vi "Measurement Logic.vi"() -> ()   [LabVIEW 2021, in "Single Tone Measurements_Class D Amplifier.lvlib"]
uses:
  Single Tone Measurements_Class D Amplifier.lvlib
  Measurement Configuration.ctl
  shared/controls/digital audio protocol/data justification.ctl
  shared/controls/digital audio protocol/endianness.ctl
  shared/controls/digital audio protocol/digital edge.ctl
  shared/controls/digital audio protocol/logic level.ctl
  shared/controls/output mode.ctl
  shared/controls/weighting filter.ctl
  shared/controls/lowpass filter.ctl
  shared/controls/highpass filter.ctl
  shared/controls/units - snr.ctl
  shared/controls/units - ratio.ctl
  Measurement Results.ctl
  <vilib>/MeasurementLink/MeasurementLink Measurement Server/Classes/MeasurementContext/MeasurementContext.lvclass
  shared/controls/single tone audio measurements.ctl
  <vilib>/PDM Acquisition Toolkit/shared/controls/clock mode.ctl
  <vilib>/PDM Acquisition Toolkit/shared/controls/PCM Frame Sync Control.ctl
  <vilib>/PDM Acquisition Toolkit/shared/controls/Digital Edge.ctl
  <vilib>/PDM Acquisition Toolkit/shared/controls/PCM Data Format Configuration.ctl
  <vilib>/PDM Acquisition Toolkit/shared/controls/PCM Bit Endianness.ctl
  <vilib>/PDM Acquisition Toolkit/shared/controls/PCM Data Justification.ctl
  shared/controls/single tone audio measurement settings.ctl
  shared/controls/audio filter settings.ctl
  shared/controls/units settings.ctl
  <vilib>/DAQmx/read.llb/DAQmx Read (Analog 1D Wfm NChan NSamp).vi
  <vilib>/PDM Acquisition Toolkit/host/API/Public/Function Generator/Configure Custom Signal (N Ch) - PCM Output Task.vi
  <vilib>/DAQmx/create/channels.llb/DAQmx Create Channel (AI-Voltage-Basic).vi
  <vilib>/DAQmx/configure/timing.llb/DAQmx Timing (Sample Clock).vi
  <vilib>/DAQmx/miscellaneous.llb/DAQmx Fill In Error Info.vi
  <vilib>/Waveform/WDTOps.llb/WDT Get Waveform Subset DBL.vi
  <vilib>/PDM Acquisition Toolkit/shared/PDM Shared.lvlib
  <vilib>/PDM Acquisition Toolkit/host/API/PDM Acquisition Toolkit.lvlib
  shared/controls/audio controls.lvlib
  shared/controls/digital audio protocol/digital audio protocol controls.lvlib
panel:
  out "results":T1={"channel"="0", "frequency (Hz)"=1000.0000024177915, "amplitude (Vrms)"=-6.256665451281146, "amplitude (dBFS)"=0.0, "SNR"=78.42395339546047, "THD+N"=-71.07176133726693, "THD"=-71.98384642729017, "dynamic range (dB)"=83.34902670182771, "gain"=-0.25666545128114626, "SFDR (dBc)"=102.93430172121762}
  out "Spectrum":cluster{"x0":dbl, "dx":dbl, "magnitude":dbl[]}(graph)={"x0"=0.0, "dx"=4.000000000559116, "magnitude"=array[6400 elements]}
  out "Waveform Graph":waveform(dbl)[](graph)=[{"t0"=timestamp(3785336549.595634 s since 1904-01-01), "dt"=1.9531249997269942e-05, "Y"=array[12800 elements], "attributes"=variant("NI_ChannelName"=variant(string "PXI1Slot4/ai0"), "NI_UnitDescription"=variant(string "Volts"))}]
  out "Bit Clock Rate":sgl=3072000.0 format="%#_6pHz"
  out "Measurement Context out":refnum<class "MeasurementContext.lvclass">
  in  "Measurement Context":refnum<class "MeasurementContext.lvclass">=refnum
  out "Measurement Results":T2={"channel name"="0", "frequency (Hz)"=1000.0000024177915, "amplitude (Vrms)"=-6.256665451281146, "amplitude (dBFS)"=0.0, "SNR"=78.42395339546047, "THD+N"=-71.07176133726693, "THD"=-71.98384642729017, "dynamic range (dB)"=83.34902670182771, "gain"=-0.25666545128114626, "SFDR (dBc)"=102.93430172121762, "output power (W)"=0.0, "wfm - t0"=0.0, "wfm - dt"=1.9531249997269942e-05, "wfm - data"=array[12800 elements], "fft - f0"=0.0, "fft - df"=4.000000000559116, "fft - data"=array[6400 elements]}
  in  "Measurement Configuration":T3={"digital channel list"="7821\\PCMo 8", "frame clock rate"=48000.0, "number of channels"=2, "channel length"=32, "bit depth"=24, "data justification"=enum."Left Justified", "endianness"=enum."MSB First", "bit clock edge sync"=enum."Rising", "frame sync edge for channel 0"=enum."Rising", "channel 0 offset"=1, "master clock channel list"="7821\\PCMo 0", "master clock rate"=12288000.0, "logic level"=enum."3.3 V", "signal frequency"=1000.0, "output mode"=enum."Power", "output level (dB)"=-1.0, "output power (W)"=1.0, "output range (pk-pk)"=15.0, "load impedance"=4.0, "signal phase"=0.0, "acq sampling rate"=51200.0, "min measurement cycles"=20, "min measurement time (s)"=0.1, "min settling cycles"=0, "min settling time (s)"=0.0, "acq channel"="PXI1Slot4/ai0", "band start"=20.0, "band stop"=20000.0, "weighting filter"=enum."Linear", "lowpass filter"=enum."No filter", "highpass filter"=enum."DC", "SNR units"=enum."dB", "THDN units"=enum."dB", "THD units"=enum."dB", "gain units"=enum."dB", "testDBL"=0.0} {"channel 0 offset" format="%#_6p"; "output power (W)" format="%0.2f"; "load impedance" format="%0.2f"; "acq sampling rate" format="%0.2f"; "frame clock rate" format="%#_6pHz"}
  out "error out":errorcluster
  in  "error in":errorcluster
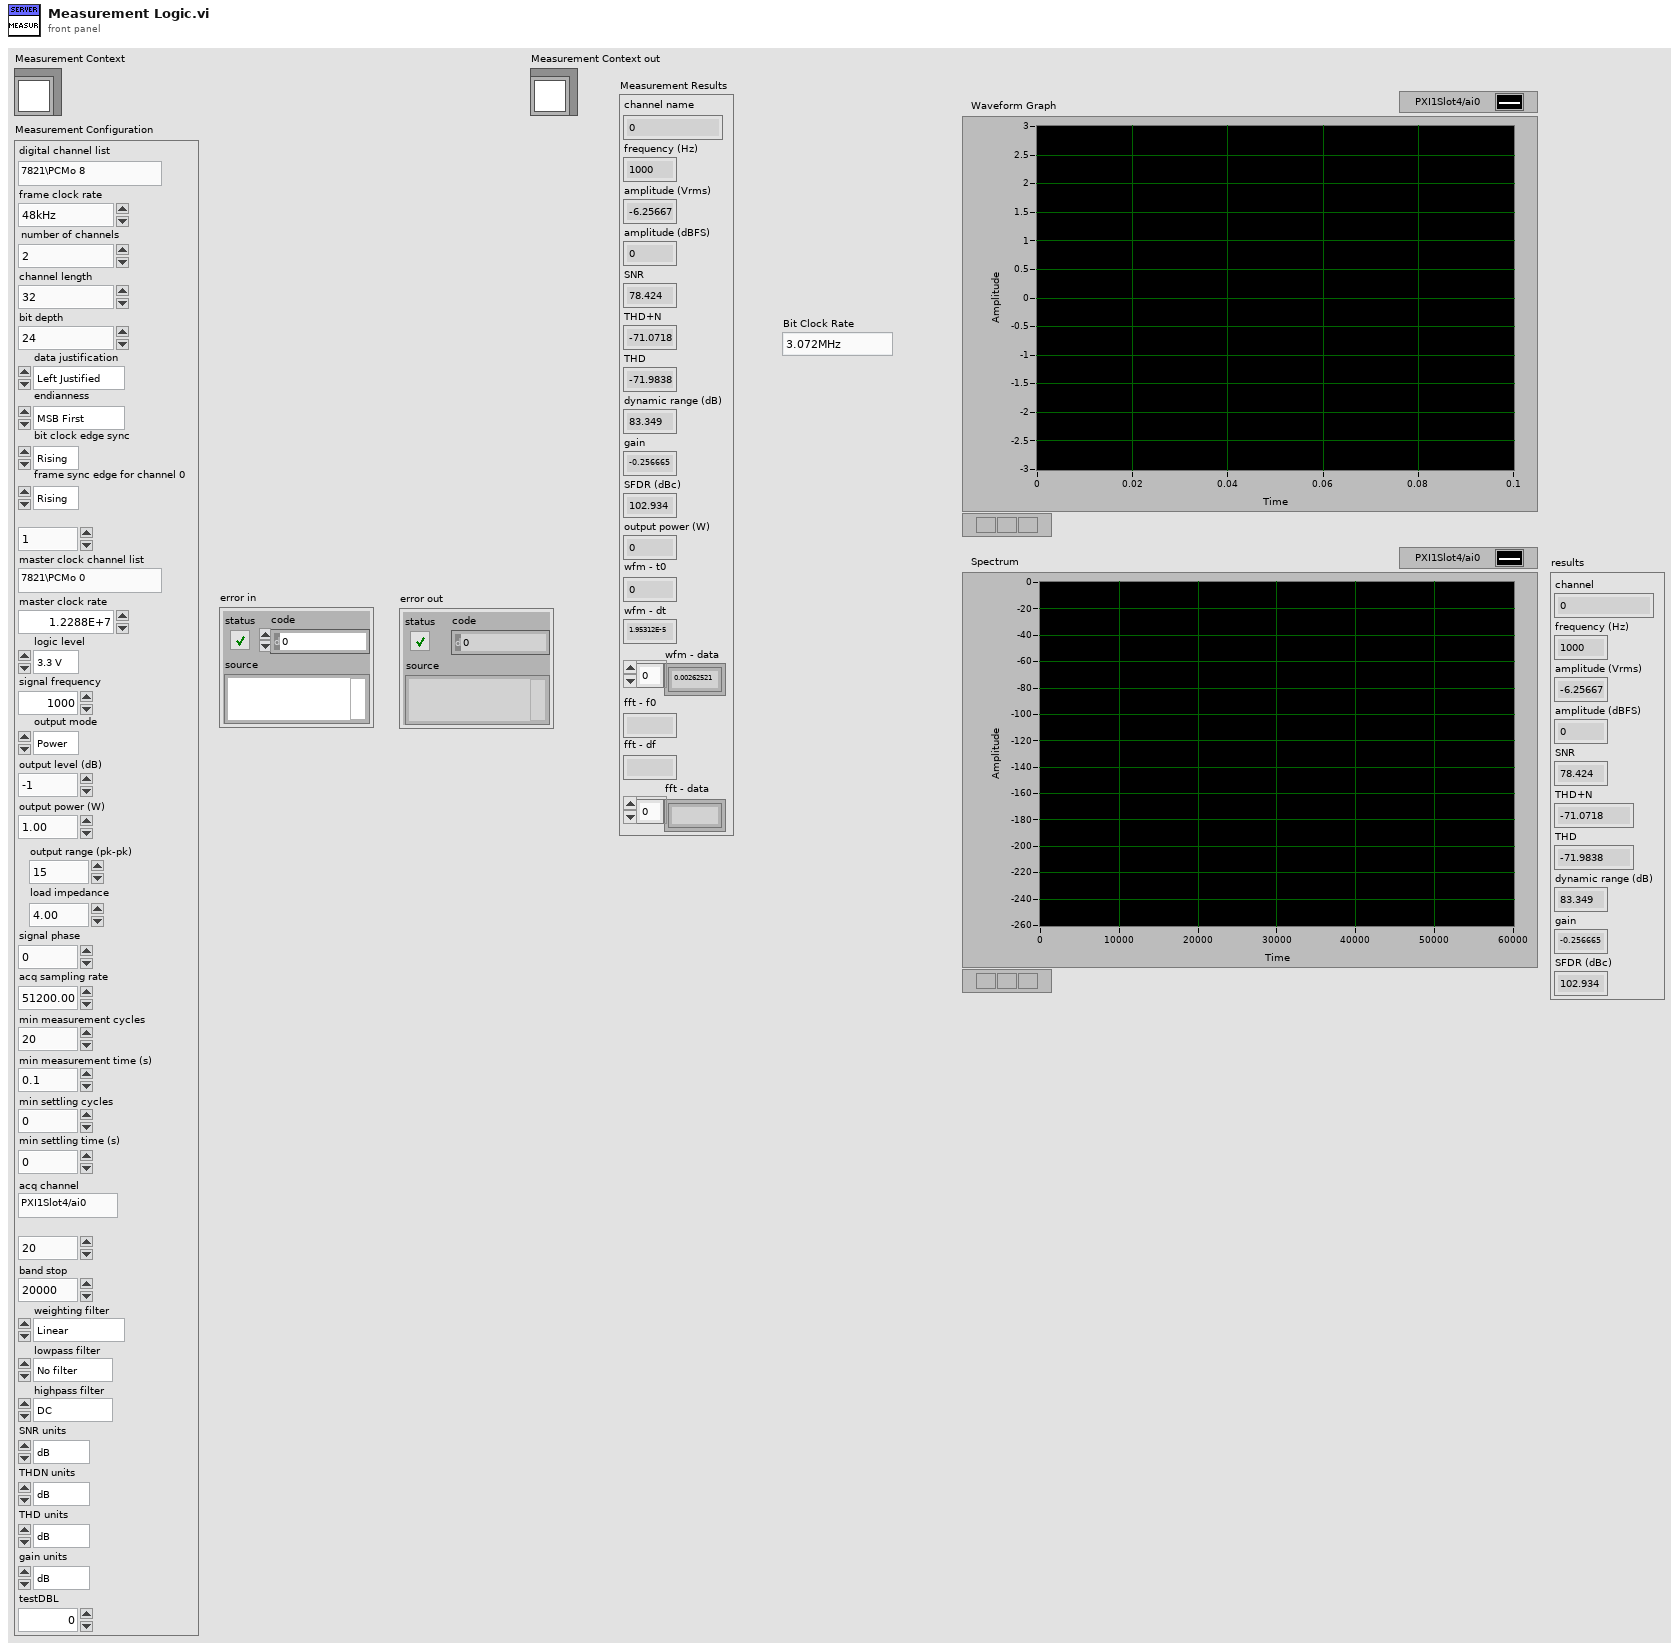
[diagram p1: front panel]
types:
  T1 = typedef "audio controls.lvlib/single tone audio measurements.ctl" = cluster{"channel":string, "frequency (Hz)":dbl, "amplitude (Vrms)":dbl, "amplitude (dBFS)":dbl, "SNR":dbl, "THD+N":dbl, "THD":dbl, "dynamic range (dB)":dbl, "gain":dbl, "SFDR (dBc)":dbl}
  T2 = typedef "Single Tone Measurements_Class D Amplifier.lvlib/Measurement Results.ctl" = cluster{"channel name":string, "frequency (Hz)":dbl, "amplitude (Vrms)":dbl, "amplitude (dBFS)":dbl, "SNR":dbl, "THD+N":dbl, "THD":dbl, "dynamic range (dB)":dbl, "gain":dbl, "SFDR (dBc)":dbl, "output power (W)":dbl, "wfm - t0":dbl, "wfm - dt":dbl, "wfm - data":dbl[], "fft - f0":dbl, "fft - df":dbl, "fft - data":dbl[]}
  T3 = typedef "Single Tone Measurements_Class D Amplifier.lvlib/Measurement Configuration.ctl" = cluster{"digital channel list":string, "frame clock rate":dbl, "number of channels":u32, "channel length":u32, "bit depth":u32, "data justification":T4, "endianness":T5, "bit clock edge sync":T6, "frame sync edge for channel 0":T6, "channel 0 offset":u32, "master clock channel list":string, "master clock rate":dbl, "logic level":T7, "signal frequency":dbl, "output mode":T8, "output level (dB)":dbl, "output power (W)":dbl, "output range (pk-pk)":dbl, "load impedance":dbl, "signal phase":dbl, "acq sampling rate":dbl, "min measurement cycles":u32, "min measurement time (s)":dbl, "min settling cycles":u32, "min settling time (s)":dbl, "acq channel":string, "band start":dbl, "band stop":dbl, "weighting filter":T9, "lowpass filter":T10, "highpass filter":T11, "SNR units":T12, "THDN units":T13, "THD units":T13, "gain units":T13, "testDBL":dbl}
  T4 = typedef "digital audio protocol controls.lvlib/data justification.ctl" = enum32{"Left Justified", "Right Justified"}
  T5 = typedef "digital audio protocol controls.lvlib/endianness.ctl" = enum32{"MSB First", "LSB First"}
  T6 = typedef "digital audio protocol controls.lvlib/digital edge.ctl" = enum32{"Rising", "Falling"}
  T7 = typedef "digital audio protocol controls.lvlib/logic level.ctl" = enum32{"3.3 V", "1.8 V", "1.2 V"}
  T8 = typedef "audio controls.lvlib/output mode.ctl" = enum32{"Level", "Power"}
  T9 = typedef "audio controls.lvlib/weighting filter.ctl" = enum32{"Linear", "A-weighting", "B-weighting", "C-weighting"}
  T10 = typedef "audio controls.lvlib/lowpass filter.ctl" = enum32{"No filter", "AES17 20kHz", "AES17 40kHz"}
  T11 = typedef "audio controls.lvlib/highpass filter.ctl" = enum32{"DC", "AC"}
  T12 = typedef "audio controls.lvlib/units - snr.ctl" = enum16{"dB", "x/y"}
  T13 = typedef "audio controls.lvlib/units - ratio.ctl" = enum16{"dB", "%", "x/y"}
  T14 = typedef "audio controls.lvlib/units settings.ctl" = cluster{"SNR units":T12, "THD+N units":T13, "THD units":T13, "gain units":T13}
  T15 = typedef "audio controls.lvlib/audio filter settings.ctl" = cluster{"weighting filter":T9, "highpass filter":T11, "lowpass filter ":T10}
  T16 = typedef "audio controls.lvlib/single tone audio measurement settings.ctl" = cluster{"Band start":dbl, "Band stop":dbl, "Amplitude":dbl, "Frequency":dbl, "Full scale range":dbl, "Channel name":string}
  T17 = typedef "PDM Shared.lvlib/PCM Data Format Configuration.ctl" = cluster{"Frame Sync Edge for Channel 0":T18, "Channel Count Per Frame":u8, "Channel Length":u16, "Bit Depth":u8, "Channel 0 Offset":u16, "Endianness":T19, "Data Justification":T20}
  T18 = typedef "PDM Shared.lvlib/Digital Edge.ctl" = enum8{"Rising", "Falling"}
  T19 = typedef "PDM Shared.lvlib/PCM Bit Endianness.ctl" = enum16{"MSB First", "LSB First"}
  T20 = typedef "PDM Shared.lvlib/PCM Data Justification.ctl" = enum16{"Left Justified", "Right Justified"}
  T21 = typedef "PDM Shared.lvlib/PCM Frame Sync Control.ctl" = cluster{"Frame Length":u16, "Frame Sync Pulse Width":u16, "Bit Clock Edge  Sync":T18}
  T22 = typedef "PDM Shared.lvlib/clock mode.ctl" = enum16{"divided clock", "DDS"}
  T23 = typedef "PDM Acquisition Class Library.lvlib/PCM Output Task.lvclass/PCM Output Task DVR.ctl" = refnum<data-value>
  T24 = typedef "PDM Acquisition Class Library.lvlib/I2S Output Task.lvclass/SignalProperties.ctl" = cluster{"cyclic signal":dbl[], "channel parameters":T25[]}
  T25 = typedef "PDM Acquisition Class Library.lvlib/I2S Output Channel.lvclass/GenerationChannelProperties.ctl" = cluster{"cyclic period":dbl, "cyclic phase offset":dbl, "gain":dbl}
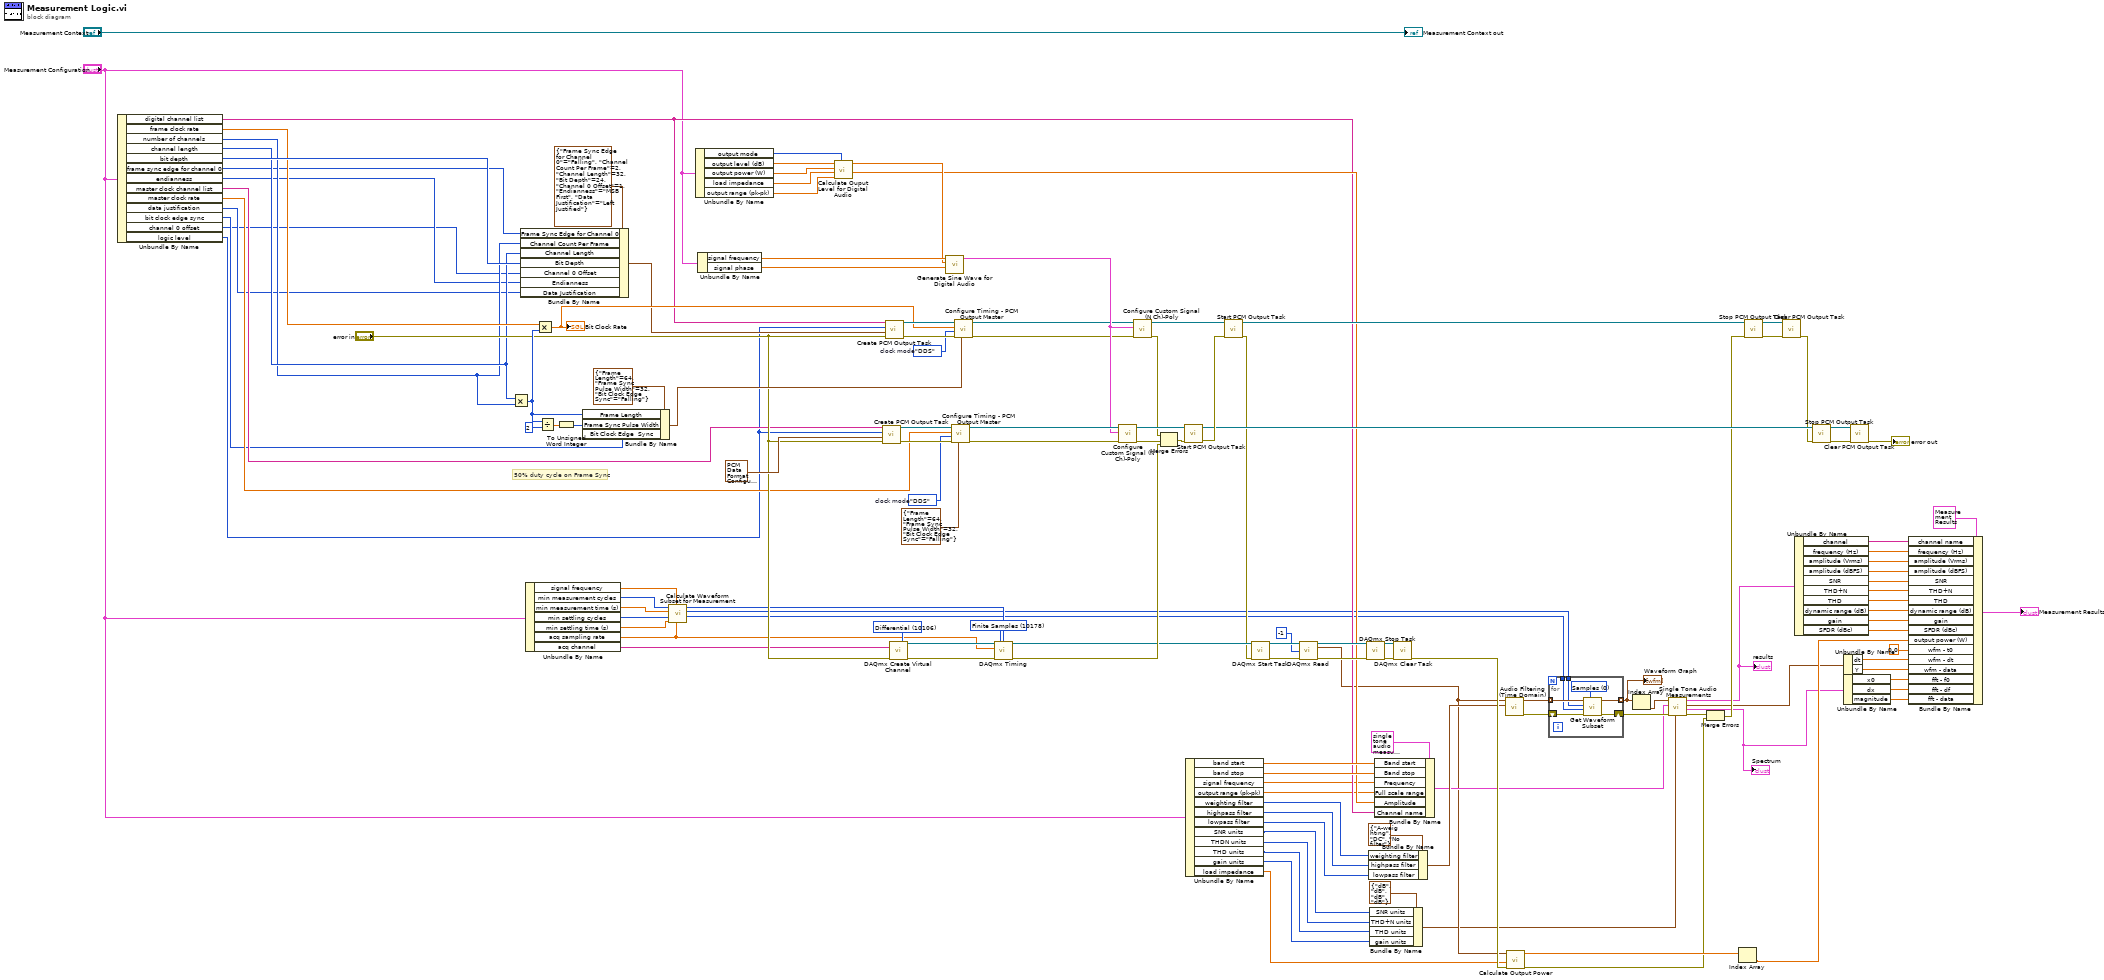
[diagram p0: block diagram]
diagram:
  w67 = 10106 items=["Default"=-1, "RSE"=10083, "NRSE"=10078, "Differential"=10106, "Pseudodifferential"=12529] ("input terminal configuration")
  w89 = 10178 items=["Finite Samples"=10178, "Continuous Samples"=10123, "Hardware Timed Single Point"=12522] ("sample mode")
  w126 = clock_mode."DDS"  # clock mode
  w129 = clock_mode."DDS"  # clock mode
  # "50% duty cycle on Frame Sync"
  n1 = Unbundle By Name("Measurement Configuration") -> ("digital channel list"=w24:string, "frame clock rate"=w72:dbl, "number of channels"=w70:u32, "channel length"=w71:u32, "bit depth"=w73:u32, "frame sync edge for channel 0"=w64:T6, "endianness"=w63:T5, "master clock channel list"=w69:string, "master clock rate"=w68:dbl, "data justification"=w65:T4, "bit clock edge sync"=w62:T6, "channel 0 offset"=w61:u32, "logic level"=w60:T7)
  n2 = Multiply(x=w71, y=w70) -> (x*y=w112:u32)
  n3 = Bundle By Name(cluster=T17 {"Frame Sync Edge for Channel 0"=enum."Falling", "Channel Count Per Frame"=2, "Channel Length"=32, "Bit Depth"=24, "Channel 0 Offset"=1, "Endianness"=enum."MSB First", "Data Justification"=enum."Left Justified"} ("PCM Data Configuration"), "Frame Sync Edge for Channel 0"=w64, "Channel Count Per Frame"=w70, "Channel Length"=w71, "Bit Depth"=w73, "Channel 0 Offset"=w61, "Endianness"=w63, "Data Justification"=w65) -> (w109:T17)
  n4 = Unbundle By Name("Measurement Configuration") -> ("signal frequency"=w16:dbl, "min measurement cycles"=w21:u32, "min measurement time (s)"=w20:dbl, "min settling cycles"=w19:u32, "min settling time (s)"=w18:dbl, "acq sampling rate"=w13:dbl, "acq channel"=w14:string)
  n5 = Multiply(x=w72, y=w112) -> (x*y=w111:dbl)
  "Bit Clock Rate" <- w111
  n6 = Divide(x=w112, y=u16 2) -> (x/y=w114:dbl)
  n7 = To Unsigned Word Integer(number=w114) -> (unsigned 16bit integer=w113:u16)
  n8 = Bundle By Name(cluster=T21 {"Frame Length"=64, "Frame Sync Pulse Width"=32, "Bit Clock Edge  Sync"=enum."Falling"} ("Frame Sync Clock Control"), "Frame Length"=w112, "Frame Sync Pulse Width"=w113, "Bit Clock Edge  Sync"=w62) -> (w116:T21)
  n9 = call "Calculate Waveform Subset for Measurement.vi"("sampling rate"=w13, "signal frequency"=w16, "minimum settling duration"=w18, "minimum settling cycles"=w19, "minimum measurement duration"=w20, "minimum measurement cycles"=w21) -> ("duration (samples)"=w10:u32, "start (samples)"=w11:u32, "total acquisition (samples)"=w12:u32)  [unwired: 3 in]
  n10 = Unbundle By Name("Measurement Configuration") -> ("output mode"=w47:T8, "output level (dB)"=w46:dbl, "output power (W)"=w45:dbl, "load impedance"=w44:dbl, "output range (pk-pk)"=w43:dbl)
  n11 = Unbundle By Name("Measurement Configuration") -> ("signal frequency"=w51:dbl, "signal phase"=w59:dbl)
  n12 = call "Calculate Ouput Level for Digital Audio.vi"("output mode"=w47, "output range (pk-pk)"=w43, "load impedance"=w44, "output power (W)"=w45, "output level (dB)"=w46) -> ("amplitude (pk)"=w25:dbl, "gain"=w50:dbl)  [unwired: 5 in]
  n13 = call <vilib>:"Create PCM Output Task.vi"("error in"="error in", "PCM data configuration"=T17 {"Frame Sync Edge for Channel 0"=enum."Falling", "Channel Count Per Frame"=2, "Channel Length"=32, "Bit Depth"=24, "Channel 0 Offset"=1, "Endianness"=enum."MSB First", "Data Justification"=enum."Left Justified"} ("PCM Data Configuration 2"), "logic level"=w60, "channel list"=w69) -> ("error out"=w127:errorcluster, "PCM output task out"=w128:T23)  [unwired: 6 in]
  n14 = call <vilib>:"Create PCM Output Task.vi"("error in"="error in", "PCM data configuration"=w109, "logic level"=w60, "channel list"=w24) -> ("error out"=w130:errorcluster, "PCM output task out"=w131:T23)  [unwired: 6 in]
  n15 = call-poly <vilib>:"DAQmx Create Virtual Channel.vi"("input terminal configuration"=w67, "physical channels"=w14, "error in"="error in") -> ("task out"=w99:refnum<k21>, "error out"=w100:errorcluster)  [unwired: 11 in]
  n16 = call "Generate Sine Wave for Digital Audio.vi"("phase"=w59, "gain"=w50, "frequency"=w51) -> ("Signal Properties"=w58:T24)  [unwired: 8 in]
  n17 = call <vilib>:"Configure Timing - PCM Output Master.vi"("Frame Sync Clock Control"=T21 {"Frame Length"=64, "Frame Sync Pulse Width"=32, "Bit Clock Edge  Sync"=enum."Falling"} ("Frame Sync Clock Control 2"), "error in"=w127, "clock mode"=w126, "Bit Clock rate"=w68, "PCM output task in"=w128) -> ("error out"=w108:errorcluster, "PCM output task out"=w107:T23)  [unwired: 4 in, 1 out]
  n18 = call <vilib>:"Configure Timing - PCM Output Master.vi"("Frame Sync Clock Control"=w116, "error in"=w130, "clock mode"=w129, "Bit Clock rate"=w111, "PCM output task in"=w131) -> ("error out"=w48:errorcluster, "PCM output task out"=w49:T23)  [unwired: 4 in, 1 out]
  n19 = call-poly <vilib>:"DAQmx Timing.vi"("task/channels in"=w99, "sample mode"=w89, "samples per channel"=w12, "rate"=w13, "error in"=w100) -> ("task out"=w90:refnum<k21>, "error out"=w91:errorcluster)  [unwired: 9 in]
  n20 = call-poly <vilib>:"Configure Custom Signal (N Ch)-Poly.vi"("error in"=w108, "signal parameters"=w58, "PCM output task in"=w107) -> ("error out"=w103:errorcluster, "PCM output task out"=w106:T23)  [unwired: 7 in]
  n21 = call-poly <vilib>:"Configure Custom Signal (N Ch)-Poly.vi"("error in"=w48, "signal parameters"=w58, "PCM output task in"=w49) -> ("error out"=w104:errorcluster, "PCM output task out"=w105:T23)  [unwired: 7 in]
  n22 = Merge Errors(w104, w103, w91) -> (w122:errorcluster)
  n23 = call <vilib>:"Start PCM Output Task.vi"("error in"=w122, "PCM output task in"=w106) -> ("error out"=w123:errorcluster, "PCM output task out"=w119:T23)  [unwired: 8 in]
  n24 = Unbundle By Name("Measurement Configuration") -> ("band start"=w33:dbl, "band stop"=w32:dbl, "signal frequency"=w22:dbl, "output range (pk-pk)"=w23:dbl, "weighting filter"=w30:T9, "highpass filter"=w29:T11, "lowpass filter"=w28:T10, "SNR units"=w5:T12, "THDN units"=w4:T13, "THD units"=w3:T13, "gain units"=w2:T13, "load impedance"=w6:dbl)
  n25 = call <vilib>:"Start PCM Output Task.vi"("error in"=w123, "PCM output task in"=w105) -> ("error out"=w66:errorcluster, "PCM output task out"=w102:T23)  [unwired: 8 in]
  n26 = call <vilib>:"DAQmx Start Task.vi"("task/channels in"=w90, "error in"=w66) -> ("task out"=w94:refnum<k21>, "error out"=w97:errorcluster)  [unwired: 12 in]
  n27 = call-poly <vilib>:"DAQmx Read.vi"("task/channels in"=w94, "number of samples per channel"=-1, "error in"=w97) -> ("task out"=w93:refnum<k21>, "data"=w15:waveform(dbl)[], "error out"=w96:errorcluster)  [unwired: 10 in]
  n28 = call <vilib>:"DAQmx Stop Task.vi"("task/channels in"=w93, "error in"=w96) -> ("task out"=w98:refnum<k21>, "error out"=w95:errorcluster)  [unwired: 12 in]
  n29 = Bundle By Name(cluster=T15 {"weighting filter"=enum."A-weighting", "highpass filter"=enum."DC", "lowpass filter "=enum."No filter"} ("filter settings"), "weighting filter"=w30, "highpass filter"=w29, "lowpass filter"=w28) -> (w27:T15)
  n30 = Bundle By Name(cluster=T14 {"SNR units"=enum."dB", "THD+N units"=enum."dB", "THD units"=enum."dB", "gain units"=enum."dB"} ("units settings"), "SNR units"=w5, "THD+N units"=w4, "THD units"=w3, "gain units"=w2) -> (w7:T14)
  n31 = Bundle By Name(cluster=T16 {"Band start"=20.0, "Band stop"=20000.0, "Amplitude"=-1.0, "Frequency"=1000.0, "Full scale range"=15.0, "Channel name"="0L"} ("measurement settings"), "Band start"=w33, "Band stop"=w32, "Frequency"=w22, "Full scale range"=w23, "Amplitude"=w25, "Channel name"=w24) -> (w26:T16)
  n32 = call <vilib>:"DAQmx Clear Task.vi"("task in"=w98, "error in"=w95) -> ("error out"=w54:errorcluster)  [unwired: 13 in]
  n33 = call "Audio Filtering (Time Domain).vi"("waveforms"=w15, "filter settings"=w27) -> ("time domain"=w40:waveform(dbl)[], "error out"=w41:errorcluster)  [unwired: 7 in]
  n34 = call "Calculate Output Power.vi"("error in (no error)"=w54, "load impedance"=w6, "waveforms"=w15) -> ("error out"=w52:errorcluster, "output power"=w57:dbl[])  [unwired: 7 in]
  n35 = for {
    tunnel: w40 -> [w143] mode=indexing
    tunnel: [w142] -> w1 mode=indexing
    shift-right: [w139] -> w39
    shift-left: w41 -> [w140]
    tunnel: w11 -> [w138]
    tunnel: w10 -> [w137]
    w141 = u16 0 items=["Samples", "Relative Time"] ("start/duration format")
    n36 = call-poly <vilib>:"Get Waveform Subset.vi"("start/duration format"=w141, "error in (no error)"=w140, "duration"=w137, "start samples/time"=w138, "waveform in"=w143) -> ("error out"=w139:errorcluster, "waveform out"=w142:waveform(dbl))  [unwired: 1 in, 2 out]
  }
  "Waveform Graph" <- w1
  n37 = Index Array(array=w1) -> (element=w42:waveform(dbl))  [unwired: 1 in]
  n38 = call "Single Tone Audio Measurements.vi"("units settings"=w7, "error in"=w39, "measurement settings"=w26, "waveform"=w42) -> ("error out"=w38:errorcluster, "spectrum"=w35:cluster{"x0":dbl, "dx":dbl, "magnitude":dbl[]}, "time domain"=w36:waveform(dbl), "results"=w37:T1)  [unwired: 4 in]
  "Spectrum" <- w35
  "results" <- w37
  n39 = Merge Errors(w38, w52) -> (w53:errorcluster)
  n40 = Index Array(array=w57) -> (element=w55:dbl)  [unwired: 1 in]
  n41 = call <vilib>:"Stop PCM Output Task.vi"("error in"=w53, "PCM output task In"=w102) -> ("error out"=w133:errorcluster, "PCM output task out"=w132:T23)  [unwired: 8 in]
  n42 = call <vilib>:"Clear PCM Output Task.vi"("error in"=w133, "PCM output task in"=w132) -> ("error out"=w118:errorcluster)  [unwired: 9 in]
  n43 = Unbundle By Name(w37) -> ("channel"=w87:string, "frequency (Hz)"=w86:dbl, "amplitude (Vrms)"=w85:dbl, "amplitude (dBFS)"=w84:dbl, "SNR"=w9:dbl, "THD+N"=w83:dbl, "THD"=w82:dbl, "dynamic range (dB)"=w81:dbl, "gain"=w80:dbl, "SFDR (dBc)"=w79:dbl)
  n44 = call <vilib>:"Stop PCM Output Task.vi"("error in"=w118, "PCM output task In"=w119) -> ("error out"=w121:errorcluster, "PCM output task out"=w120:T23)  [unwired: 8 in]
  n45 = Unbundle By Name(w36) -> ("dt"=w78:dbl, "Y"=w77:dbl[])
  n46 = Unbundle By Name(w35) -> ("x0"=w76:dbl, "dx"=w75:dbl, "magnitude"=w74:dbl[])
  n47 = call <vilib>:"Clear PCM Output Task.vi"("error in"=w121, "PCM output task in"=w120) -> ("error out"=→"error out":errorcluster)  [unwired: 9 in]
  n48 = Bundle By Name(cluster=T2 {"channel name"="", "frequency (Hz)"=0.0, "amplitude (Vrms)"=0.0, "amplitude (dBFS)"=0.0, "SNR"=0.0, "THD+N"=0.0, "THD"=0.0, "dynamic range (dB)"=0.0, "gain"=0.0, "SFDR (dBc)"=0.0, "output power (W)"=0.0, "wfm - t0"=0.0, "wfm - dt"=0.0, "wfm - data"=[], "fft - f0"=0.0, "fft - df"=0.0, "fft - data"=[]} ("Measurement Results"), "channel name"=w87, "frequency (Hz)"=w86, "amplitude (Vrms)"=w85, "amplitude (dBFS)"=w84, "SNR"=w9, "THD+N"=w83, "THD"=w82, "dynamic range (dB)"=w81, "gain"=w80, "SFDR (dBc)"=w79, "output power (W)"=w55, "wfm - t0"=0.0, "wfm - dt"=w78, "wfm - data"=w77, "fft - f0"=w76, "fft - df"=w75, "fft - data"=w74) -> (→"Measurement Results":T2)
  "Measurement Context out" <- "Measurement Context"
